vi "ADC SNR_Sweep.vi"(8 "error in (no error)":errorcluster, 9 "Sequence parameters":string[][](array[string])=[["Min limit", "Max limit", "Register sheet file", "Register Sheet"], ["", "", "CC2600.xls", "TX_BLE;Trim"], ["Reg write (addr;value)", "Operating frequency [Hz]", "", ""], ["NA", "2.44G", "", ""]], 10 "Run type":i32, 11 "Method parameters":T3={"Dev"={"Do not disturb DUT"=FALSE, "XOSC"=32000000.0, "Board type"="", "EM"="", "Configure tempboard"=TRUE, "Device specific info"=[], "Generic Object"=refnum}, "Method"={"Run type"=1, "Test name"="Current LPM2 4", "Comment"="", "Results folder"="", "AFC"=enum."Off", "Method name"="Current LPM2 4", "Method results"={"Excel brief report"=FALSE, "Spotfire report"=FALSE, "Starfish report"=FALSE}, "Operator"="", "Reference time"=timestamp(0 s since 1904-01-01), "AFC delay"=0.0, "Initialization"=enum."Enabled", "MD5 Sum"="", "HW addon board"=enum."None", "AFC Regsheet"="", "AFC Regfile"=path "", "dummy"=0.0}, "Inst"={"Instr"={"PS1"={"Name"="", "GPIB address"="", "VISA session"=""}, "PS2"={"Name"="", "GPIB address"="", "VISA session"=""}, "TC1"={"Name"="", "GPIB address"="", "VISA session"=""}, "TC2"={"Name"="", "GPIB address"="", "VISA session"=""}, "SA1"={"Name"="", "GPIB address"="", "VISA session"=""}, "SA2"={"Name"="", "GPIB address"="", "VISA session"=""}, "SG1"={"Name"="", "GPIB address"="", "VISA session"=""}, "SG2"={"Name"="", "GPIB address"="", "VISA session"=""}, "SG3"={"Name"="", "GPIB address"="", "VISA session"=""}, "MI1"={"Name"="", "GPIB address"="", "VISA session"=""}, "MI2"={"Name"="", "GPIB address"="", "VISA session"=""}, "SW SA"={"Name"="", "Controller addr"=""}, "SW SG"={"Name"="", "Controller addr"=""}, "MI3"={"Name"="", "GPIB address"="", "VISA session"=""}}, "Switchbox"={"RF Path"=0, "Cal compensation"=enum."TX", "Switchbox gain mode"="", "State"=enum."TX"}, "Instr to control (i.e. SA1)"="Default", "Intrument info string"=""}, "Sequence parameters"=[["Weight", "Min Limit", "Max Limit", "Register Sheet", "", "", "", "", "", "", "", "", ""], ["Vital", "", "1", "LPM2", "", "", "", "", "", "", "", "", ""], ["Resolution", "Reg write (addr;value)", "Chip mode", "Range", "", "", "", "", "", "", "", "", ""], ["u", "NA", "", "auto", "", "", "", "", "", "", "", "", ""]], "Cond"={"Temp logged"=25.0, "VDD1_PS1_6V"=-999.0, "VDD2_PS1_25V"=-999.0, "VDD4_PS2_25V"=-999.0, "VDD3_PS2_6V"=-999.0}, "Meas config"={"X-axis inner loop index"=32000000, "Y-axis outer loop index"=32000000, "X-axis"=[], "Y-axis"=[], "X-axis array req size"=32000000, "Y-axis array req size"=32000000, "Param description"=[], "Use meas clust for reporting"=FALSE, "Parameter index (page)"=0, "X-axis name"="", "Y-axis name"=""}} {"Cond"."VDD3_PS2_6V" format="%.3f"; "Cond"."VDD4_PS2_25V" format="%.3f"; "Cond"."VDD2_PS1_25V" format="%.3f"; "Cond"."VDD1_PS1_6V" format="%.3f"; "Method"."dummy" format="%.1p"; "Method"."AFC delay" format="%.1p"; "Dev"."XOSC" format="%.3p"}) -> (0 "error out":errorcluster, 1 "End method error":T1, 2 "Short Results":string[](array[string]), 3 "Result summary":string[][](array[string])=[["Critical", "Output Power@2405 MHz", "-3", "4", "dBm"], ["Critical", "Output Power@2410 MHz", "-3", "4", "dBm"]])   [LabVIEW 2019]
doc: "[AutoDocStart]Performs crystal accuracy measurements. Measures the offset from ideal frequency. Primarily used for tuning XOSC capacitors and verifying XOSC trims.\n\nSweeping parameters: operating frequency, OSC override value and VDDR level\n\nResults: Offset frequency in ppm[AutoDocEnd]"
uses:
  User Lib/Utilities/Cluster definitions/Method input.ctl
  User Lib/Utilities/Cluster definitions/Device specific info.ctl
  User Lib/Utilities/Controls/Automatic Frequency Compensation types.ctl
  User Lib/Utilities/Controls/Method Reports.ctl
  User Lib/Utilities/Cluster definitions/Method Initialization.ctl
  User Lib/Utilities/Controls/HW addon boards.ctl
  User Lib/Utilities/Cluster definitions/Instr clust.ctl
  User Lib/Utilities/Switchbox control/SwitchBox_State._ENUMctl.ctl
  User Lib/Utilities/Cluster definitions/End method error cluster.ctl
  d1e189ac-5c6c-49e1-a56b-a93f7ba1e5c3.vi
  89ac9e08-f822-48c3-bf7b-b9620a48f2c1.vi
  afbe0b8a-4628-4f4a-a689-fb3560c1b1a6.vi
  160c279e-5860-4c4e-a522-43dd8a66307b.vi
  eb3a7dab-0138-448e-bc0a-4bb49588a4f1.vi
  4ae92598-944e-459b-8fa7-3a23a971f601.vi
  e1f832d6-75bf-4ba2-931c-48c142ce58ac.vi
  User Lib/Utilities/Cluster definitions/DUT VDD4.ctl
  User Lib/Utilities/Cluster definitions/DUT VDD3.ctl
  User Lib/Utilities/Cluster definitions/DUT VDD2.ctl
  User Lib/Utilities/Cluster definitions/DUT VDD1.ctl
  User Lib/Utilities/Cluster definitions/DUT vdd control.ctl
panel:
  in  "Tab Control":T2(tab)
  # "°C"
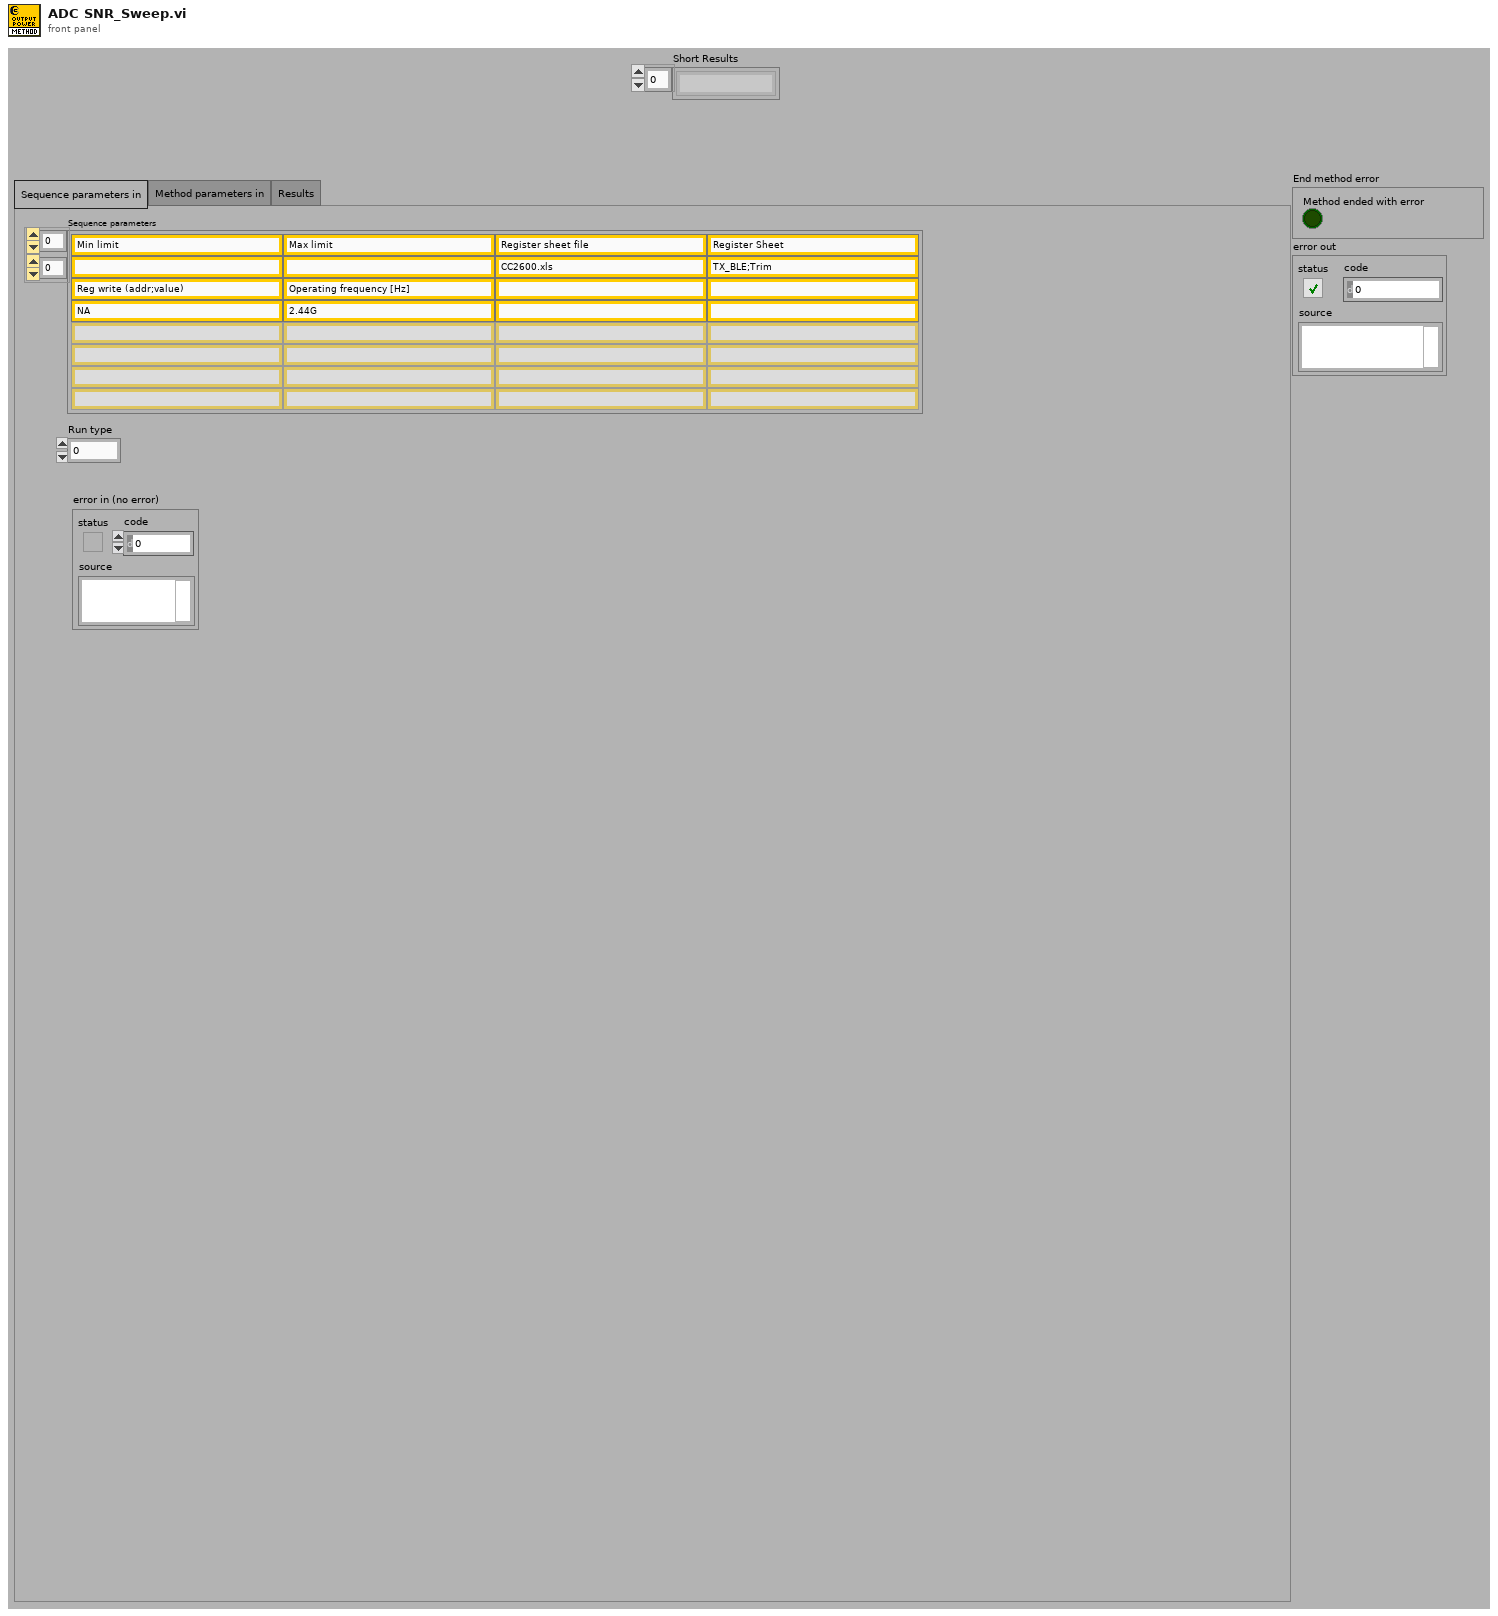
[diagram p1: front panel]
types:
  T1 = typedef "End method error cluster.ctl" = cluster{"Method ended with error":bool}
  T2 = enum32{"Sequence parameters in", "Method parameters in", "Results"}
  T3 = typedef "Method input.ctl" = cluster{"Dev":cluster{"Do not disturb DUT":bool, "XOSC":dbl, "Board type":string, "EM":string, "Configure tempboard":bool, "Device specific info":T4[], "Generic Object":refnum<class>}, "Method":cluster{"Run type":i32, "Test name":string, "Comment":string, "Results folder":string, "AFC":T5, "Method name":string, "Method results":T6, "Operator":string, "Reference time":timestamp, "AFC delay":dbl, "Initialization":T7, "MD5 Sum":string, "HW addon board":T8, "AFC Regsheet":string, "AFC Regfile":path, "dummy":dbl}, "Inst":T9, "Sequence parameters":string[][], "Cond":cluster{"Temp logged":dbl, "VDD1_PS1_6V":dbl, "VDD2_PS1_25V":dbl, "VDD4_PS2_25V":dbl, "VDD3_PS2_6V":dbl}, "Meas config":cluster{"X-axis inner loop index":i32, "Y-axis outer loop index":i32, "X-axis":string[], "Y-axis":string[], "X-axis array req size":i32, "Y-axis array req size":i32, "Param description":string[][], "Use meas clust for reporting":bool, "Parameter index (page)":i32, "X-axis name":string, "Y-axis name":string}}
  T4 = typedef "Device specific info.ctl" = cluster{"EM number":u8, "IP address":string, "Enabled":bool, "Slot no":u8, "RF path":u8, "EM name":string, "Wafer info":string, "AFC frequency ppm":dbl, "Register writes":string[][], "Meas data":string[][][], "Device comment":string}
  T5 = typedef "Automatic Frequency Compensation types.ctl" = enum16{"Off", "Compensate Instrument frequency", "Compensate DUT frequency", "Predictive - Compensate Instrument frequency", "Predictive - Compensate DUT frequency", "Do not skip re-init - Compensate Instrument frequency", "Do not skip re-init - Compensate DUT frequency"}
  T6 = typedef "Method Reports.ctl" = cluster{"Excel brief report":bool, "Spotfire report":bool, "Starfish report":bool}
  T7 = typedef "Method Initialization.ctl" = enum16{"Enabled", "Skip Instr and Device Init", "Enabled with Separate Flash", "Set PS, Device Init and Skip Instr Init", "Skip Device Init"}
  T8 = typedef "HW addon boards.ctl" = enum16{"None", "Current meas 5EM", "Stresstest 10EM"}
  T9 = typedef "Instr clust.ctl" = cluster{"Instr":cluster{"PS1":cluster{"Name":string, "GPIB address":string, "VISA session":refnum<visa-resource-name>}, "PS2":cluster{"Name":string, "GPIB address":string, "VISA session":refnum<visa-resource-name>}, "TC1":cluster{"Name":string, "GPIB address":string, "VISA session":refnum<visa-resource-name>}, "TC2":cluster{"Name":string, "GPIB address":string, "VISA session":refnum<visa-resource-name>}, "SA1":cluster{"Name":string, "GPIB address":string, "VISA session":refnum<visa-resource-name>}, "SA2":cluster{"Name":string, "GPIB address":string, "VISA session":refnum<visa-resource-name>}, "SG1":cluster{"Name":string, "GPIB address":string, "VISA session":refnum<visa-resource-name>}, "SG2":cluster{"Name":string, "GPIB address":string, "VISA session":refnum<visa-resource-name>}, "SG3":cluster{"Name":string, "GPIB address":string, "VISA session":refnum<visa-resource-name>}, "MI1":cluster{"Name":string, "GPIB address":string, "VISA session":refnum<visa-resource-name>}, "MI2":cluster{"Name":string, "GPIB address":string, "VISA session":refnum<visa-resource-name>}, "SW SA":cluster{"Name":string, "Controller addr":string}, "SW SG":cluster{"Name":string, "Controller addr":string}, "MI3":cluster{"Name":string, "GPIB address":string, "VISA session":refnum<visa-resource-name>}}, "Switchbox":cluster{"RF Path":i32, "Cal compensation":enum16{"TX", "RX", "Interferer", "No compensation", "Interferer2"}, "Switchbox gain mode":string, "State":T10}, "Instr to control (i.e. SA1)":string, "Intrument info string":string}
  T10 = typedef "SwitchBox_State._ENUMctl.ctl" = enum16{"TX", "RX", "SP:TX", "SP:RX", "SW:TX", "SW:RX"}
  T11 = typedef "DUT vdd control.ctl" = cluster{"VDD4 config":T12, "VDD3 config":T13, "VDD2 config":T14, "VDD1 config":T15}
  T12 = typedef "DUT VDD4.ctl" = u16
  T13 = typedef "DUT VDD3.ctl" = u16
  T14 = typedef "DUT VDD2.ctl" = u16
  T15 = typedef "DUT VDD1.ctl" = u16
  T16 = cluster{"Fundamental Frequency":dbl, "Sampling Frequncy":dbl, "No of Harmonics":u8, "Window":enum16{"None ", "Hanning", "Hamming", "Blackman-Harris", "Exact Blackman", "Blackman", "Flat Top", "4 Term B-Harris ", "7 Term B-Harris"}, "Blackman (fundamental power) bins)":dbl}
  T17 = enum32{"NI Card Settings", "Memory Read Setting", "DC Capture", "ADC Ramp", "ADC Sine", "SNR", "Cap Calibration"}
  T18 = enum32{"Read from Memory", "Read .dat file", "NI Card Capture", "None"}
  T19 = cluster{"Path to Save plot":path, "Path to Raw Data plot":path}
  T20 = cluster{"Save INL/DNL Plot(Ramp)":bool, "Save SNR Plot":bool, "Save INL/DNL Plot(Sine)":bool, "Save INL/DNL Raw Data(Ramp)":bool, "Save SNR Raw Data":bool, "Save INL/DNL Raw Data(Sine)":bool, "Save DC Raw data":bool, "Save  Raw Data(Sine)":bool}
  T21 = cluster{"SNR":dbl, "SNRD":dbl, "THD":dbl, "ENOB (SNRD)":dbl, "SFDR":dbl, "ENOB (SNR)":dbl, "Noise Power":dbl, "Signal power":dbl}
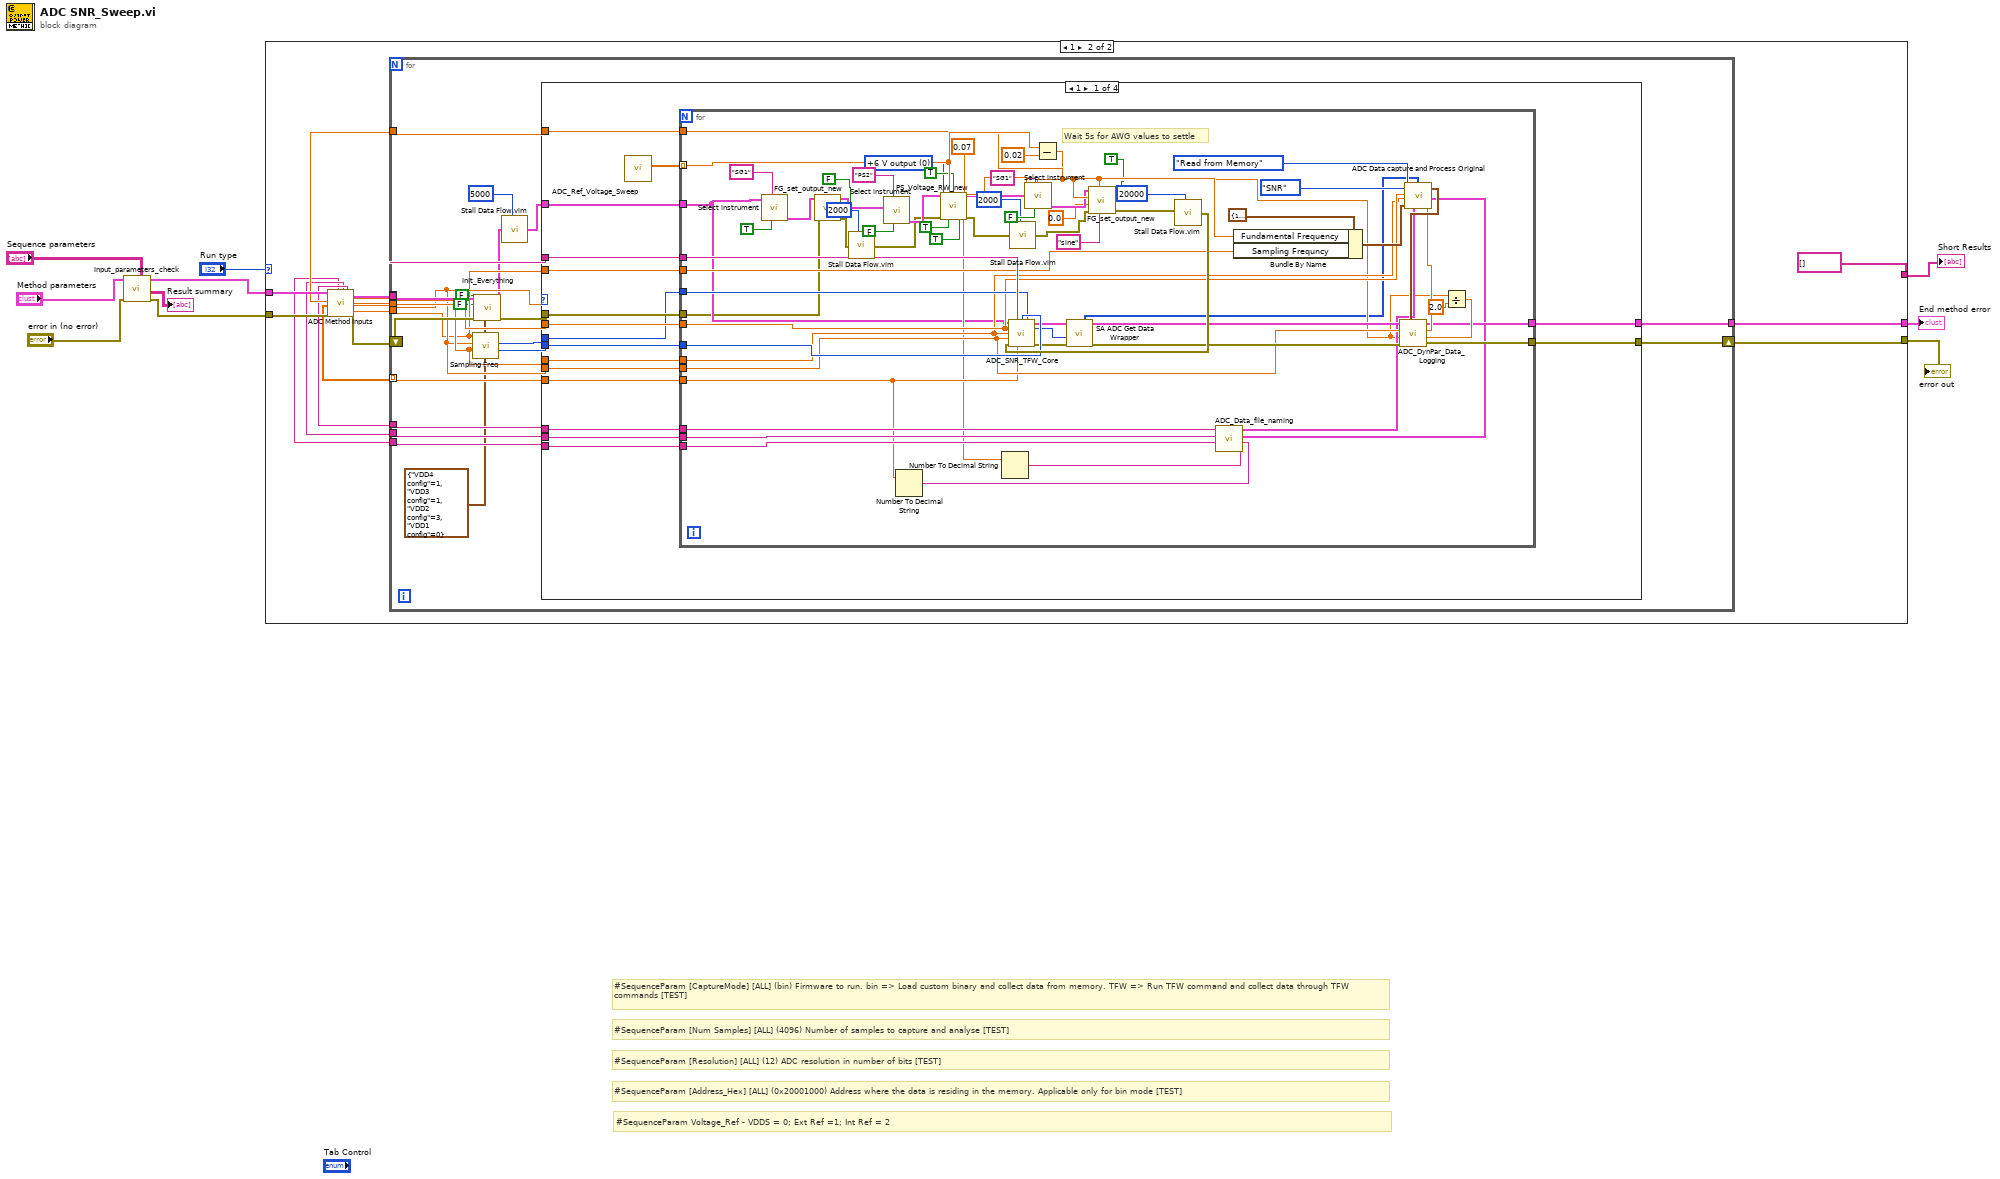
[diagram p0: block diagram]
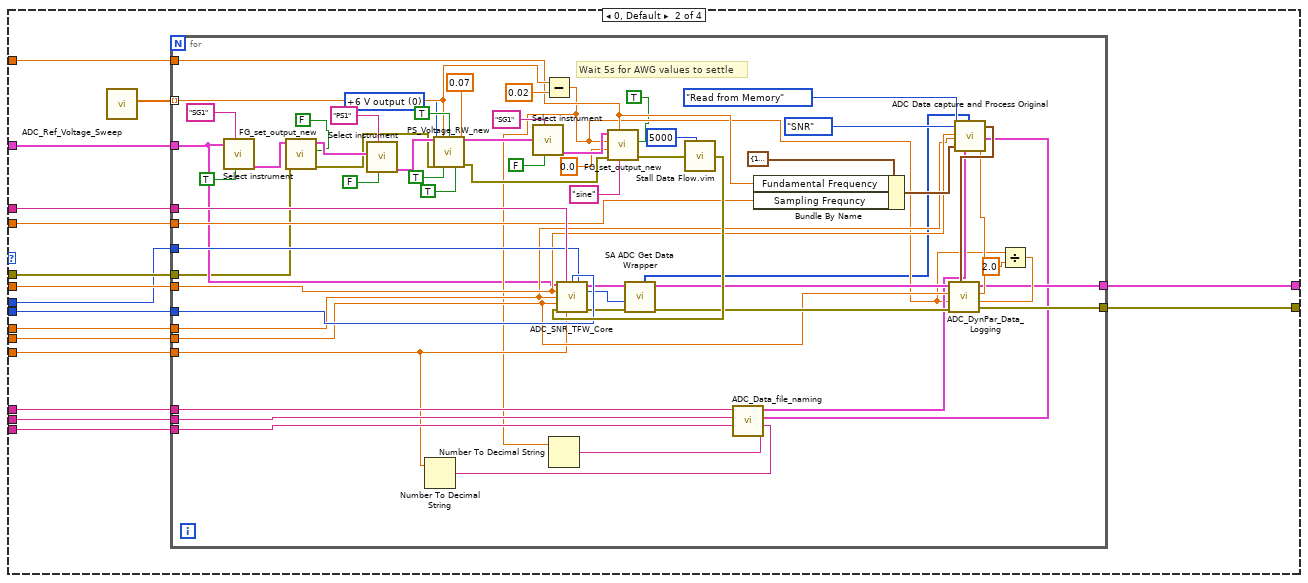
[diagram p3: hidden frame]
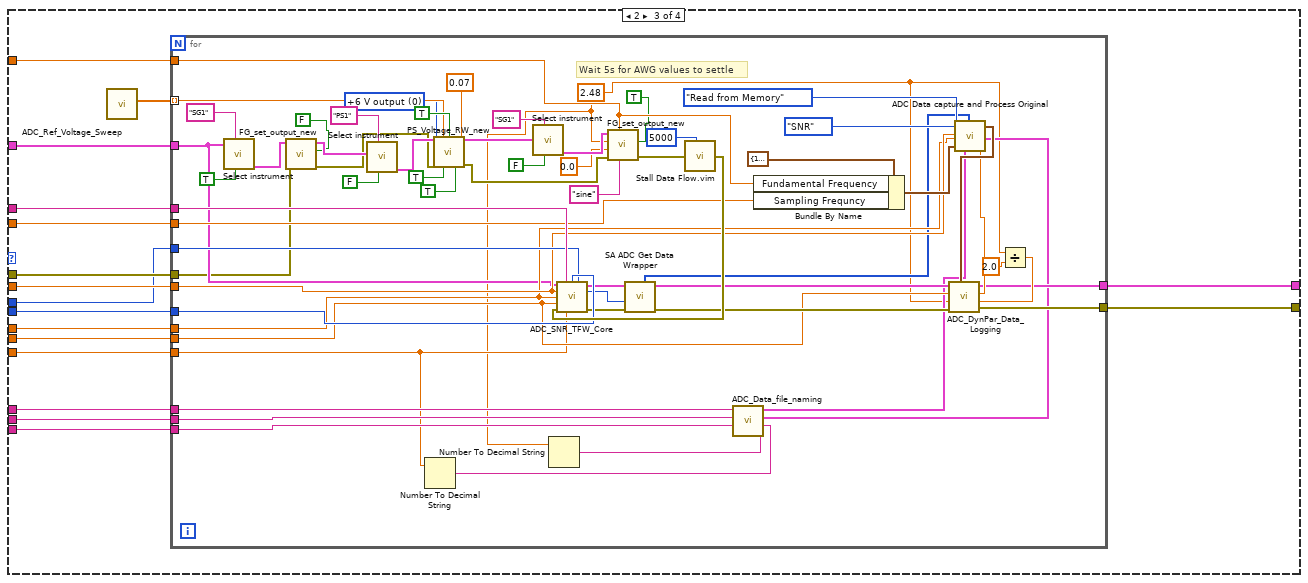
[diagram p4: hidden frame]
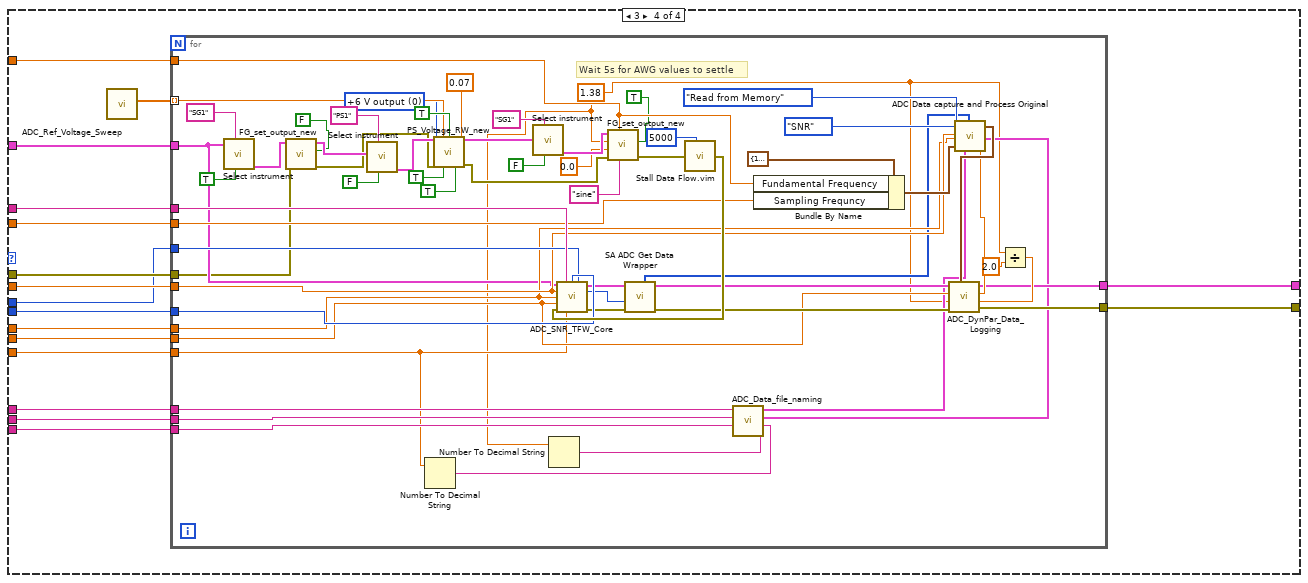
[diagram p5: hidden frame]
diagram:
  # "#SequenceParam Voltage_Ref - VDDS = 0; Ext Ref =1; Int Ref = 2"
  # "#SequenceParam [Num Samples] [ALL] (4096) Number of samples to capture and analyse [TEST]"
  # "#SequenceParam [CaptureMode] [ALL] (bin) Firmware to run. bin => Load custom binary and collect data from memory. TFW => Run TFW command and collect data through TFW commands [TEST]"
  # "#SequenceParam [Address_Hex] [ALL] (0x20001000) Address where the data is residing in the memory. Applicable only for bin mode [TEST]"
  # "#SequenceParam [Resolution] [ALL] (12) ADC resolution in number of bits [TEST]"
  n1 = call "Input_parameters_check.vi"("Sequence parameters"="Sequence parameters", "error in"="error in (no error)", "Method cluster in"="Method parameters") -> ("error out"=w10:errorcluster, "Result summary"=→"Result summary":string[][], "Method cluster out"=w6:T3)  [unwired: 6 in]
  n2 = case shown="1" "Run type" {
    tunnel: w10 -> [w11 w28]
    tunnel: w6 -> [_ w27]
    tunnel: [string[] [] string[] []] -> w3
    tunnel: [w11 w18] -> w2
    tunnel: [_ w17] -> w1
    frame 0, Default {
      # "Run type 0 is only for formatting the result summary"
    }
    frame 1 {
      n3 = call "ADC Method Inputs.vi"("Method cluster in"=w27, "error in (no error)"=w28) -> ("Capture Mode"=w21:string, "Signal Freq"=w20:dbl, "ADC Chnl No."=w13:dbl[], "Sampling Freq String"=w14:string, "Resolution String"=w15:string, "Voltage Ref String"=w16:string, "Method cluster out"=w26:T3, "Num Samples"=w24:dbl, "Resolution"=w23:dbl, "Voltage Ref"=w22:dbl, "Sampling Freq"=w19:dbl, "error out"=w25:errorcluster)  [unwired: 6 in]
      n4 = for {
        tunnel: w26 -> [w52]
        tunnel: w24 -> [w49]
        tunnel: w23 -> [w48]
        tunnel: w22 -> [w47]
        tunnel: w21 -> [w46]
        tunnel: w20 -> [w43]
        tunnel: w19 -> [w42]
        tunnel: [w40] -> w17
        tunnel: w16 -> [w39]
        tunnel: w15 -> [w38]
        tunnel: w14 -> [w37]
        shift-right: [w41] -> w18
        shift-left: w25 -> [w51]
        tunnel: w13 -> [w36] mode=indexing
        n5 = call "Sampling Freq.vi"("Resolution"=w48, "Voltage Ref"=w47, "Sampling Freq"=w42) -> ("LGPT Count"=w45:u16, "SCOMP"=w44:u16)  [unwired: 7 in]
        n6 = call "Init_Everything.vi"("VDD config"=T11 {"VDD4 config"=1, "VDD3 config"=1, "VDD2 config"=3, "VDD1 config"=0}, "error in"=w51, "Support current measurement?"=FALSE, "Override VDD Config"=FALSE, "Method cluster In"=w52) -> ("error out"=w50:errorcluster, "Method cluster out"=w34:T3)  [unwired: 3 in, 2 out]
        n7 = call "Stall Data Flow.vim"("value in"=w34, "milliseconds to wait"=u32 5000) -> ("value out"=w35:T3)  [unwired: 1 out]
        n8 = case shown="1" w47 {
          tunnel: w35 -> [w68 w151 w230 w308]
          tunnel: w50 -> [w67 w150 w229 w307]
          tunnel: w49 -> [w66 w149 w228 w306]
          tunnel: w48 -> [w65 w148 w227 w305]
          tunnel: w47 -> [w64 w147 w226 w304]
          tunnel: w46 -> [w63 w146 w225 w303]
          tunnel: w45 -> [w62 w145 w224 w302]
          tunnel: w44 -> [w61 w144 w223 w301]
          tunnel: w43 -> [w60 w143 w222 w300]
          tunnel: w36 -> [w59 w142 w221 w299]
          tunnel: w42 -> [w58 w141 w220 w298]
          tunnel: [w57 w140 w219 w297] -> w40
          tunnel: [w56 w139 w218 w296] -> w41
          tunnel: w39 -> [w55 w138 w217 w295]
          tunnel: w38 -> [w54 w137 w216 w294]
          tunnel: w37 -> [w53 w136 w215 w293]
          frame 1 {
            n9 = call "ADC_Ref_Voltage_Sweep.vi"() -> ("Ref voltage sweep"=w69:dbl[])  [unwired: 11 in]
            n10 = for {
              tunnel: w69 -> [w129] mode=indexing
              tunnel: w68 -> [w98]
              tunnel: w67 -> [w97]
              tunnel: w66 -> [w119]
              tunnel: w65 -> [w118]
              tunnel: w64 -> [w113]
              tunnel: w63 -> [w132]
              tunnel: w62 -> [w131]
              tunnel: w61 -> [w130]
              tunnel: w60 -> [w122]
              tunnel: w59 -> [w103]
              tunnel: w58 -> [w121]
              tunnel: [w110] -> w57
              tunnel: [w109] -> w56
              tunnel: w55 -> [w106]
              tunnel: w54 -> [w105]
              tunnel: w53 -> [w104]
              w76 = u16 0 items=["+6 V output", "+25 V output", "-25 V output", "ALL TERM"] ("Output Terminals")
              # "Wait 5s for AWG values to settle"
              n11 = call "Select instrument.vi"("Method cluster (T) / Instr cluster (F)"=TRUE, "Instr.Instr to control (i.e. SA1)"="SG1", "Method cluster in"=w98) -> ("Instr out"=w82:T9)  [unwired: 6 in, 2 out]
              n12 = call "FG_set_output_new.vi"("Enable Output?"=FALSE, "error in"=w97, "InstrCluster in"=w82) -> ("error out"=w75:errorcluster, "InstrCluster out"=w80:T9)  [unwired: 7 in]
              n13 = call "Stall Data Flow.vim"("value in"=w75, "milliseconds to wait"=u32 2000) -> ("value out"=w74:errorcluster)  [unwired: 1 out]
              n14 = call "Select instrument.vi"("Method cluster (T) / Instr cluster (F)"=FALSE, "Instr.Instr to control (i.e. SA1)"="PS2", "Instr in"=w80) -> ("Instr out"=w87:T9)  [unwired: 6 in, 2 out]
              n15 = Number To Decimal String(number=w103) -> (decimal integer string=w102:string)  [unwired: 1 in]
              n16 = call "PS_Voltage_RW_new.vi"("InstrCluster in"=w87, "Set Voltage"=w129, "Limit to 4V (T)"=TRUE, "Current(0)"=0.07, "Output Terminals"=w76, "error in (no error)"=w74, "Off (F)                         On (T)"=TRUE, "Read (F)                      Write (T)"=TRUE) -> ("InstrCluster out"=w88:T9, "error out"=w72:errorcluster)  [unwired: 5 in, 1 out]
              n17 = call "Stall Data Flow.vim"("value in"=w72, "milliseconds to wait"=u32 2000) -> ("value out"=w71:errorcluster)  [unwired: 1 out]
              n18 = call "Select instrument.vi"("Method cluster (T) / Instr cluster (F)"=FALSE, "Instr.Instr to control (i.e. SA1)"="SG1", "Instr in"=w88) -> ("Instr out"=w91:T9)  [unwired: 6 in, 2 out]
              n19 = Subtract(x=w129, y=0.02) -> (x-y=w101:dbl)
              n20 = Number To Decimal String(number=w101) -> (decimal integer string=w100:string)  [unwired: 1 in]
              n21 = call "FG_set_output_new.vi"("Enable Output?"=TRUE, "Function (DC, Sine, Square, Triangle, Ramp up, Ramp down, Pulse)"="sine", "Frequency [Hz]"=w122, "error in"=w71, "Low voltage"=0.0, "High voltage (or DC)"=w101, "InstrCluster in"=w91) -> ("error out"=w134:errorcluster)  [unwired: 3 in, 1 out]
              n22 = call "Stall Data Flow.vim"("value in"=w134, "milliseconds to wait"=u32 20000) -> ("value out"=w133:errorcluster)  [unwired: 1 out]
              n23 = call "ADC_SNR_TFW_Core.vi"("Method cluster in"=w98, "Capture Mode"=w132, "LGPT Count"=w131, "SCOMP"=w130, "No. Samples"=w119, "Resolution"=w118, "Voltage Ref"=w113, "error in"=w133, "ADC Chnl No."=w103) -> ("Method cluster out 2"=w127:T3, "ResPar[0] Data Address"=w126:u32, "error out"=w128:errorcluster)  [unwired: 3 in, 1 out]
              n24 = call "SA ADC Get Data Wrapper.vi"("error in"=w128, "Data Address"=w126, "Method cluster in"=w127) -> ("error out"=w115:errorcluster, "output cluster"=w116:T3, "ADC samples"=w99:u32[])  [unwired: 3 in, 3 out]
              n25 = call "ADC_Data_file_naming.vi"("Amplitude (Vpp)"=w100, "ADC Chn. No"=w102, "Sampling Freq String"=w104, "Resolution String"=w105, "Voltage Ref String"=w106) -> ("path to save"=w107:T19, "Save data"=w108:T20)  [unwired: 5 in]
              n26 = Bundle By Name(cluster=T16 {"Fundamental Frequency"=10000.0, "Sampling Frequncy"=250000.0, "No of Harmonics"=9, "Window"=enum."7 Term B-Harris", "Blackman (fundamental power) bins)"=1.0} ("Inputs for Dyanmic para"), "Fundamental Frequency"=w122, "Sampling Frequncy"=w121) -> (w120:T16)
              n27 = call "ADC Data capture and Process Original.vi"("ADC Output Read Method"=T18."Read from Memory", "Select the Tab to project"=T17."SNR", "No.of samples(SNR)"=w119, "Resolution"=w118, "Inputs for Dyanmic para"=w120, "Save data"=w108, "Waveform"=w99, "path to save"=w107) -> ("detected Throughput"=w114:dbl, "Dynamic Parameters"=w117:T21)  [unwired: 13 in, 5 out]
              n28 = Divide(x=w101, y=2.0) -> (x/y=w111:dbl)
              n29 = call "ADC_DynPar_Data_Logging.vi"("Offset (V)"=w111, "detected Throughput"=w114, "Dynamic Parameters"=w117, "error in (no error)"=w115, "Amplitude (Vpp)"=w101, "Ref Voltage"=w113, "Method Cluster In"=w116) -> ("error out"=w109:errorcluster, "End method error"=w110:T1)  [unwired: 3 in]
            }
          }
          frame 0, Default {
            n30 = call "ADC_Ref_Voltage_Sweep.vi"() -> ("Ref voltage sweep"=w152:dbl[])  [unwired: 11 in]
            n31 = for {
              tunnel: w152 -> [w193] mode=indexing
              tunnel: w151 -> [w162]
              tunnel: w150 -> [w158]
              tunnel: w149 -> [w183]
              tunnel: w148 -> [w182]
              tunnel: w147 -> [w177]
              tunnel: w146 -> [w196]
              tunnel: w145 -> [w195]
              tunnel: w144 -> [w194]
              tunnel: w143 -> [w186]
              tunnel: w142 -> [w167]
              tunnel: w141 -> [w185]
              tunnel: [w174] -> w140
              tunnel: [w173] -> w139
              tunnel: w138 -> [w170]
              tunnel: w137 -> [w169]
              tunnel: w136 -> [w168]
              w153 = u16 0 items=["+6 V output", "+25 V output", "-25 V output", "ALL TERM"] ("Output Terminals")
              # "Wait 5s for AWG values to settle"
              n32 = call "Select instrument.vi"("Method cluster (T) / Instr cluster (F)"=TRUE, "Instr.Instr to control (i.e. SA1)"="SG1", "Method cluster in"=w162) -> ("Instr out"=w161:T9)  [unwired: 6 in, 2 out]
              n33 = call "FG_set_output_new.vi"("Enable Output?"=FALSE, "error in"=w158, "InstrCluster in"=w161) -> ("error out"=w157:errorcluster, "InstrCluster out"=w159:T9)  [unwired: 7 in]
              n34 = call "Select instrument.vi"("Method cluster (T) / Instr cluster (F)"=FALSE, "Instr.Instr to control (i.e. SA1)"="PS1", "Instr in"=w159) -> ("Instr out"=w204:T9)  [unwired: 6 in, 2 out]
              n35 = Number To Decimal String(number=w167) -> (decimal integer string=w166:string)  [unwired: 1 in]
              n36 = call "PS_Voltage_RW_new.vi"("InstrCluster in"=w204, "Set Voltage"=w193, "Limit to 4V (T)"=TRUE, "Current(0)"=0.07, "Output Terminals"=w153, "error in (no error)"=w157, "Off (F)                         On (T)"=TRUE, "Read (F)                      Write (T)"=TRUE) -> ("InstrCluster out"=w205:T9, "error out"=w206:errorcluster)  [unwired: 5 in, 1 out]
              n37 = call "Select instrument.vi"("Method cluster (T) / Instr cluster (F)"=FALSE, "Instr.Instr to control (i.e. SA1)"="SG1", "Instr in"=w205) -> ("Instr out"=w209:T9)  [unwired: 6 in, 2 out]
              n38 = Subtract(x=w193, y=0.02) -> (x-y=w165:dbl)
              n39 = Number To Decimal String(number=w165) -> (decimal integer string=w164:string)  [unwired: 1 in]
              n40 = call "FG_set_output_new.vi"("Enable Output?"=TRUE, "Function (DC, Sine, Square, Triangle, Ramp up, Ramp down, Pulse)"="sine", "Frequency [Hz]"=w186, "error in"=w206, "Low voltage"=0.0, "High voltage (or DC)"=w165, "InstrCluster in"=w209) -> ("error out"=w198:errorcluster)  [unwired: 3 in, 1 out]
              n41 = call "Stall Data Flow.vim"("value in"=w198, "milliseconds to wait"=u32 5000) -> ("value out"=w197:errorcluster)  [unwired: 1 out]
              n42 = call "ADC_SNR_TFW_Core.vi"("Method cluster in"=w162, "Capture Mode"=w196, "LGPT Count"=w195, "SCOMP"=w194, "No. Samples"=w183, "Resolution"=w182, "Voltage Ref"=w177, "error in"=w197, "ADC Chnl No."=w167) -> ("Method cluster out 2"=w191:T3, "ResPar[0] Data Address"=w190:u32, "error out"=w192:errorcluster)  [unwired: 3 in, 1 out]
              n43 = call "SA ADC Get Data Wrapper.vi"("error in"=w192, "Data Address"=w190, "Method cluster in"=w191) -> ("error out"=w179:errorcluster, "output cluster"=w180:T3, "ADC samples"=w163:u32[])  [unwired: 3 in, 3 out]
              n44 = call "ADC_Data_file_naming.vi"("Amplitude (Vpp)"=w164, "ADC Chn. No"=w166, "Sampling Freq String"=w168, "Resolution String"=w169, "Voltage Ref String"=w170) -> ("path to save"=w171:T19, "Save data"=w172:T20)  [unwired: 5 in]
              n45 = Bundle By Name(cluster=T16 {"Fundamental Frequency"=10000.0, "Sampling Frequncy"=250000.0, "No of Harmonics"=9, "Window"=enum."7 Term B-Harris", "Blackman (fundamental power) bins)"=1.0} ("Inputs for Dyanmic para"), "Fundamental Frequency"=w186, "Sampling Frequncy"=w185) -> (w184:T16)
              n46 = call "ADC Data capture and Process Original.vi"("ADC Output Read Method"=T18."Read from Memory", "Select the Tab to project"=T17."SNR", "No.of samples(SNR)"=w183, "Resolution"=w182, "Inputs for Dyanmic para"=w184, "Save data"=w172, "Waveform"=w163, "path to save"=w171) -> ("detected Throughput"=w178:dbl, "Dynamic Parameters"=w181:T21)  [unwired: 13 in, 5 out]
              n47 = Divide(x=w165, y=2.0) -> (x/y=w175:dbl)
              n48 = call "ADC_DynPar_Data_Logging.vi"("Offset (V)"=w175, "detected Throughput"=w178, "Dynamic Parameters"=w181, "error in (no error)"=w179, "Amplitude (Vpp)"=w165, "Ref Voltage"=w177, "Method Cluster In"=w180) -> ("error out"=w173:errorcluster, "End method error"=w174:T1)  [unwired: 3 in]
            }
          }
          frame 2 {
            n49 = call "ADC_Ref_Voltage_Sweep.vi"() -> ("Ref voltage sweep"=w231:dbl[])  [unwired: 11 in]
            n50 = for {
              tunnel: w231 -> [w272] mode=indexing
              tunnel: w230 -> [w242]
              tunnel: w229 -> [w238]
              tunnel: w228 -> [w262]
              tunnel: w227 -> [w261]
              tunnel: w226 -> [w256]
              tunnel: w225 -> [w275]
              tunnel: w224 -> [w274]
              tunnel: w223 -> [w273]
              tunnel: w222 -> [w265]
              tunnel: w221 -> [w246]
              tunnel: w220 -> [w264]
              tunnel: [w253] -> w219
              tunnel: [w252] -> w218
              tunnel: w217 -> [w249]
              tunnel: w216 -> [w248]
              tunnel: w215 -> [w247]
              w232 = u16 0 items=["+6 V output", "+25 V output", "-25 V output", "ALL TERM"] ("Output Terminals")
              w233 = 2.48
              # "Wait 5s for AWG values to settle"
              n51 = call "Select instrument.vi"("Method cluster (T) / Instr cluster (F)"=TRUE, "Instr.Instr to control (i.e. SA1)"="SG1", "Method cluster in"=w242) -> ("Instr out"=w241:T9)  [unwired: 6 in, 2 out]
              n52 = call "FG_set_output_new.vi"("Enable Output?"=FALSE, "error in"=w238, "InstrCluster in"=w241) -> ("error out"=w237:errorcluster, "InstrCluster out"=w239:T9)  [unwired: 7 in]
              n53 = call "Select instrument.vi"("Method cluster (T) / Instr cluster (F)"=FALSE, "Instr.Instr to control (i.e. SA1)"="PS1", "Instr in"=w239) -> ("Instr out"=w283:T9)  [unwired: 6 in, 2 out]
              n54 = Number To Decimal String(number=w246) -> (decimal integer string=w245:string)  [unwired: 1 in]
              n55 = call "PS_Voltage_RW_new.vi"("InstrCluster in"=w283, "Set Voltage"=w272, "Limit to 4V (T)"=TRUE, "Current(0)"=0.07, "Output Terminals"=w232, "error in (no error)"=w237, "Off (F)                         On (T)"=TRUE, "Read (F)                      Write (T)"=TRUE) -> ("InstrCluster out"=w284:T9, "error out"=w285:errorcluster)  [unwired: 5 in, 1 out]
              n56 = call "Select instrument.vi"("Method cluster (T) / Instr cluster (F)"=FALSE, "Instr.Instr to control (i.e. SA1)"="SG1", "Instr in"=w284) -> ("Instr out"=w288:T9)  [unwired: 6 in, 2 out]
              n57 = Number To Decimal String(number=w233) -> (decimal integer string=w244:string)  [unwired: 1 in]
              n58 = call "FG_set_output_new.vi"("Enable Output?"=TRUE, "Function (DC, Sine, Square, Triangle, Ramp up, Ramp down, Pulse)"="sine", "Frequency [Hz]"=w265, "error in"=w285, "Low voltage"=0.0, "High voltage (or DC)"=w233, "InstrCluster in"=w288) -> ("error out"=w277:errorcluster)  [unwired: 3 in, 1 out]
              n59 = call "Stall Data Flow.vim"("value in"=w277, "milliseconds to wait"=u32 5000) -> ("value out"=w276:errorcluster)  [unwired: 1 out]
              n60 = call "ADC_SNR_TFW_Core.vi"("Method cluster in"=w242, "Capture Mode"=w275, "LGPT Count"=w274, "SCOMP"=w273, "No. Samples"=w262, "Resolution"=w261, "Voltage Ref"=w256, "error in"=w276, "ADC Chnl No."=w246) -> ("Method cluster out 2"=w270:T3, "ResPar[0] Data Address"=w269:u32, "error out"=w271:errorcluster)  [unwired: 3 in, 1 out]
              n61 = call "SA ADC Get Data Wrapper.vi"("error in"=w271, "Data Address"=w269, "Method cluster in"=w270) -> ("error out"=w258:errorcluster, "output cluster"=w259:T3, "ADC samples"=w243:u32[])  [unwired: 3 in, 3 out]
              n62 = call "ADC_Data_file_naming.vi"("Amplitude (Vpp)"=w244, "ADC Chn. No"=w245, "Sampling Freq String"=w247, "Resolution String"=w248, "Voltage Ref String"=w249) -> ("path to save"=w250:T19, "Save data"=w251:T20)  [unwired: 5 in]
              n63 = Bundle By Name(cluster=T16 {"Fundamental Frequency"=10000.0, "Sampling Frequncy"=250000.0, "No of Harmonics"=9, "Window"=enum."7 Term B-Harris", "Blackman (fundamental power) bins)"=1.0} ("Inputs for Dyanmic para"), "Fundamental Frequency"=w265, "Sampling Frequncy"=w264) -> (w263:T16)
              n64 = call "ADC Data capture and Process Original.vi"("ADC Output Read Method"=T18."Read from Memory", "Select the Tab to project"=T17."SNR", "No.of samples(SNR)"=w262, "Resolution"=w261, "Inputs for Dyanmic para"=w263, "Save data"=w251, "Waveform"=w243, "path to save"=w250) -> ("detected Throughput"=w257:dbl, "Dynamic Parameters"=w260:T21)  [unwired: 13 in, 5 out]
              n65 = Divide(x=w233, y=2.0) -> (x/y=w254:dbl)
              n66 = call "ADC_DynPar_Data_Logging.vi"("Offset (V)"=w254, "detected Throughput"=w257, "Dynamic Parameters"=w260, "error in (no error)"=w258, "Amplitude (Vpp)"=w233, "Ref Voltage"=w256, "Method Cluster In"=w259) -> ("error out"=w252:errorcluster, "End method error"=w253:T1)  [unwired: 3 in]
            }
          }
          frame 3 {
            n67 = call "ADC_Ref_Voltage_Sweep.vi"() -> ("Ref voltage sweep"=w309:dbl[])  [unwired: 11 in]
            n68 = for {
              tunnel: w309 -> [w350] mode=indexing
              tunnel: w308 -> [w320]
              tunnel: w307 -> [w316]
              tunnel: w306 -> [w340]
              tunnel: w305 -> [w339]
              tunnel: w304 -> [w334]
              tunnel: w303 -> [w353]
              tunnel: w302 -> [w352]
              tunnel: w301 -> [w351]
              tunnel: w300 -> [w343]
              tunnel: w299 -> [w324]
              tunnel: w298 -> [w342]
              tunnel: [w331] -> w297
              tunnel: [w330] -> w296
              tunnel: w295 -> [w327]
              tunnel: w294 -> [w326]
              tunnel: w293 -> [w325]
              w310 = u16 0 items=["+6 V output", "+25 V output", "-25 V output", "ALL TERM"] ("Output Terminals")
              w311 = 1.38
              # "Wait 5s for AWG values to settle"
              n69 = call "Select instrument.vi"("Method cluster (T) / Instr cluster (F)"=TRUE, "Instr.Instr to control (i.e. SA1)"="SG1", "Method cluster in"=w320) -> ("Instr out"=w319:T9)  [unwired: 6 in, 2 out]
              n70 = call "FG_set_output_new.vi"("Enable Output?"=FALSE, "error in"=w316, "InstrCluster in"=w319) -> ("error out"=w315:errorcluster, "InstrCluster out"=w317:T9)  [unwired: 7 in]
              n71 = call "Select instrument.vi"("Method cluster (T) / Instr cluster (F)"=FALSE, "Instr.Instr to control (i.e. SA1)"="PS1", "Instr in"=w317) -> ("Instr out"=w361:T9)  [unwired: 6 in, 2 out]
              n72 = Number To Decimal String(number=w324) -> (decimal integer string=w323:string)  [unwired: 1 in]
              n73 = call "PS_Voltage_RW_new.vi"("InstrCluster in"=w361, "Set Voltage"=w350, "Limit to 4V (T)"=TRUE, "Current(0)"=0.07, "Output Terminals"=w310, "error in (no error)"=w315, "Off (F)                         On (T)"=TRUE, "Read (F)                      Write (T)"=TRUE) -> ("InstrCluster out"=w362:T9, "error out"=w363:errorcluster)  [unwired: 5 in, 1 out]
              n74 = call "Select instrument.vi"("Method cluster (T) / Instr cluster (F)"=FALSE, "Instr.Instr to control (i.e. SA1)"="SG1", "Instr in"=w362) -> ("Instr out"=w366:T9)  [unwired: 6 in, 2 out]
              n75 = Number To Decimal String(number=w311) -> (decimal integer string=w322:string)  [unwired: 1 in]
              n76 = call "FG_set_output_new.vi"("Enable Output?"=TRUE, "Function (DC, Sine, Square, Triangle, Ramp up, Ramp down, Pulse)"="sine", "Frequency [Hz]"=w343, "error in"=w363, "Low voltage"=0.0, "High voltage (or DC)"=w311, "InstrCluster in"=w366) -> ("error out"=w355:errorcluster)  [unwired: 3 in, 1 out]
              n77 = call "Stall Data Flow.vim"("value in"=w355, "milliseconds to wait"=u32 5000) -> ("value out"=w354:errorcluster)  [unwired: 1 out]
              n78 = call "ADC_SNR_TFW_Core.vi"("Method cluster in"=w320, "Capture Mode"=w353, "LGPT Count"=w352, "SCOMP"=w351, "No. Samples"=w340, "Resolution"=w339, "Voltage Ref"=w334, "error in"=w354, "ADC Chnl No."=w324) -> ("Method cluster out 2"=w348:T3, "ResPar[0] Data Address"=w347:u32, "error out"=w349:errorcluster)  [unwired: 3 in, 1 out]
              n79 = call "SA ADC Get Data Wrapper.vi"("error in"=w349, "Data Address"=w347, "Method cluster in"=w348) -> ("error out"=w336:errorcluster, "output cluster"=w337:T3, "ADC samples"=w321:u32[])  [unwired: 3 in, 3 out]
              n80 = call "ADC_Data_file_naming.vi"("Amplitude (Vpp)"=w322, "ADC Chn. No"=w323, "Sampling Freq String"=w325, "Resolution String"=w326, "Voltage Ref String"=w327) -> ("path to save"=w328:T19, "Save data"=w329:T20)  [unwired: 5 in]
              n81 = Bundle By Name(cluster=T16 {"Fundamental Frequency"=10000.0, "Sampling Frequncy"=250000.0, "No of Harmonics"=9, "Window"=enum."7 Term B-Harris", "Blackman (fundamental power) bins)"=1.0} ("Inputs for Dyanmic para"), "Fundamental Frequency"=w343, "Sampling Frequncy"=w342) -> (w341:T16)
              n82 = call "ADC Data capture and Process Original.vi"("ADC Output Read Method"=T18."Read from Memory", "Select the Tab to project"=T17."SNR", "No.of samples(SNR)"=w340, "Resolution"=w339, "Inputs for Dyanmic para"=w341, "Save data"=w329, "Waveform"=w321, "path to save"=w328) -> ("detected Throughput"=w335:dbl, "Dynamic Parameters"=w338:T21)  [unwired: 13 in, 5 out]
              n83 = Divide(x=w311, y=2.0) -> (x/y=w332:dbl)
              n84 = call "ADC_DynPar_Data_Logging.vi"("Offset (V)"=w332, "detected Throughput"=w335, "Dynamic Parameters"=w338, "error in (no error)"=w336, "Amplitude (Vpp)"=w311, "Ref Voltage"=w334, "Method Cluster In"=w337) -> ("error out"=w330:errorcluster, "End method error"=w331:T1)  [unwired: 3 in]
            }
          }
        }
      }
    }
  }
  "Short Results" <- w3
  "End method error" <- w1
  "error out" <- w2
